vi "Get Ports.vi"(8 "error in (no error)":errorcluster, 11 "configuration file path":path=path "C:/UTP/config/Configuration.ini") -> (0 "error out":errorcluster, 2 "Devices":string[](array[string]), 3 "Ports":u32[](array[numeric]))   [LabVIEW 2023]
uses:
  <vilib>/Utility/config.llb/NI_LVConfig.lvlib
  <vilib>/Utility/config.llb/Read Key (U32).vi
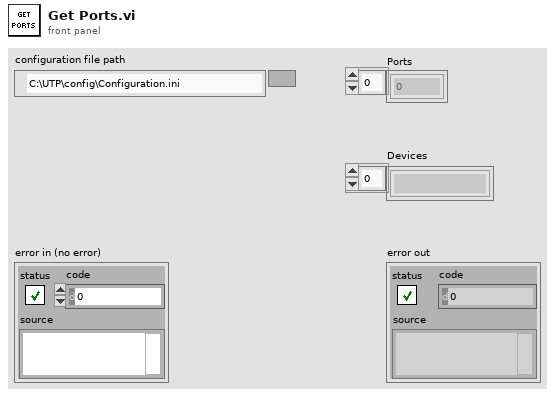
[diagram p1: front panel]
types:
  T1 = typedef "NI_LVConfig.lvlib/Config Data RefNum.ctl" = refnum<k1>
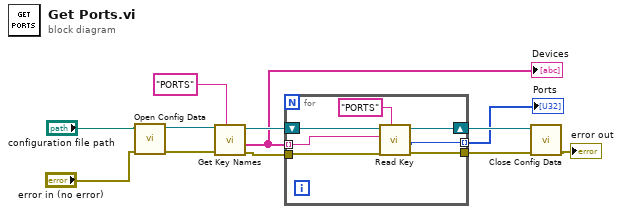
[diagram p0: block diagram]
diagram:
  n1 = call <vilib>:"Open Config Data.vi"("error in (no error)"="error in (no error)", "configuration file path"="configuration file path") -> ("error out"=w8:errorcluster, "refnum"=w11:T1)  [unwired: 7 in, 1 out]
  n2 = call <vilib>:"Get Key Names.vi"("section"="PORTS", "error in (no error)"=w8, "refnum"=w11) -> ("error out"=w7:errorcluster, "key names"=w4:string[], "refnum out"=w10:T1)  [unwired: 5 in, 1 out]
  "Devices" <- w4
  n3 = for {
    shift-right: [w18] -> w9
    shift-left: w10 -> [w19]
    tunnel: w4 -> [w17] mode=indexing
    tunnel: w7 -> [w16]
    tunnel: [w15] -> w6
    tunnel: [w14] -> w1 mode=indexing
    n4 = call-poly <vilib>:"Read Key.vi"("section"="PORTS", "error in (no error)"=w16, "key"=w17, "refnum"=w19) -> ("error out"=w15:errorcluster, "value"=w14:u32, "refnum out"=w18:T1)  [unwired: 4 in, 1 out]
  }
  "Ports" <- w1
  n5 = call <vilib>:"Close Config Data.vi"("error in (no error)"=w6, "refnum"=w9) -> ("error out"=→"error out":errorcluster)  [unwired: 8 in, 1 out]
